vi "FRCts20_WebMethods_S3Upload.vi"(8 "error in (no error)":errorcluster, 9 "Bucket":string, 10 "Object Path":string, 11 "Temporary URL":string) -> (0 "error out":errorcluster)   [LabVIEW 2014, in "FRCts20_Backend_Engine.lvlib"]
uses:
  Backend/source/VI Source/FRCts20_Backend_Engine.lvlib
  <vilib>/National Instruments/NI Amazon Web Services (AWS) Toolkit for LabVIEW/S3/vi source/Typedefs/AMZ_S3_AWS Credentials.ctl
  <vilib>/National Instruments/NI Amazon Web Services (AWS) Toolkit for LabVIEW/S3/vi source/Typedefs/AMZ_S3_API_POST Multipart Object Request Parameters.ctl
  <vilib>/National Instruments/NI Amazon Web Services (AWS) Toolkit for LabVIEW/S3/vi source/Typedefs/AMZ_S3_ACL.ctl
  <vilib>/National Instruments/NI Amazon Web Services (AWS) Toolkit for LabVIEW/S3/vi source/Typedefs/AMZ_S3_Storage Class.ctl
  <vilib>/National Instruments/NI Amazon Web Services (AWS) Toolkit for LabVIEW/S3/vi source/Typedefs/AMZ_S3_Object Metadata.ctl
  <vilib>/National Instruments/NI Amazon Web Services (AWS) Toolkit for LabVIEW/S3/vi source/LV Interface for Amazon S3.lvlib
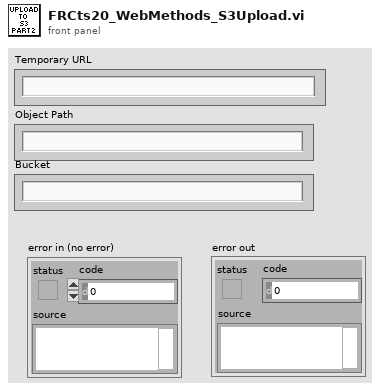
[diagram p1: front panel]
types:
  T1 = typedef "LV Interface for Amazon S3.lvlib/AMZ_S3_API_POST Multipart Object Request Parameters.ctl" = cluster{"Content Type":string, "ACL":T2, "Storage Class":T3, "User Metadata":T4[]}
  T2 = typedef "LV Interface for Amazon S3.lvlib/AMZ_S3_ACL.ctl" = enum16{"private", "public-read", "public-read-write", "authenticated-read", "bucket-owner-read", "bucket-owner-full-control"}
  T3 = typedef "LV Interface for Amazon S3.lvlib/AMZ_S3_Storage Class.ctl" = enum16{"STANDARD", "REDUCED_REDUNDANCY"}
  T4 = typedef "LV Interface for Amazon S3.lvlib/AMZ_S3_Object Metadata.ctl" = cluster{"Key":string, "Value":string}
  T5 = typedef "LV Interface for Amazon S3.lvlib/AMZ_S3_AWS Credentials.ctl" = cluster{"Access Key":string, "Secret Key":string}
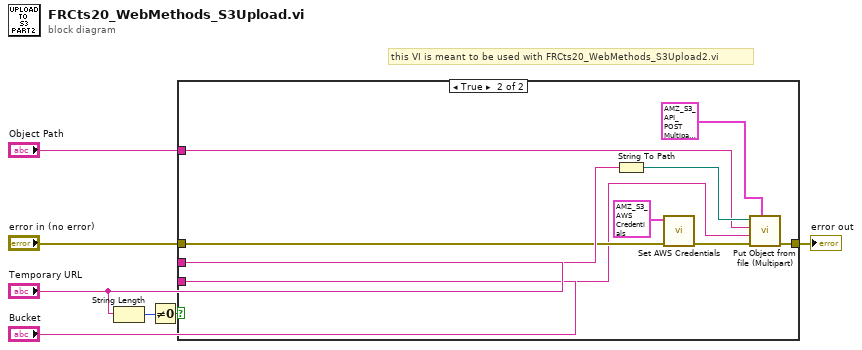
[diagram p0: block diagram]
diagram:
  # "this VI is meant to be used with FRCts20_WebMethods_S3Upload2.vi"
  n1 = String Length(string="Temporary URL") -> (length=w4:i32)
  n2 = Not Equal To 0?(x=w4) -> (x != 0?=w1:bool)
  n3 = case shown="True" w1 {
    tunnel: [w8 w17] -> w7
    tunnel: "Temporary URL" -> [_ w16]
    tunnel: "Object Path" -> [_ w10]
    tunnel: "error in (no error)" -> [w8 w11]
    tunnel: "Bucket" -> [_ w9]
    frame False {
    }
    frame True {
      n4 = String To Path(string=w16) -> (path=w13:path)
      n5 = call <vilib>:"Set AWS Credentials.vi"("error in (no error)"=w11, "AWS Credentials in"=T5 {"Access Key"="AKIAIBWID7GQA3ZVLBGQ", "Secret Key"="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"}) -> ("error out"=w15:errorcluster)  [unwired: 9 in]
      n6 = call <vilib>:"Put Object from file (Multipart).vi"("Request Parameters"=T1 {"Content Type"="binary/octet-stream", "ACL"=enum."public-read", "Storage Class"=enum."REDUCED_REDUNDANCY", "User Metadata"=[]}, "error in (no error)"=w15, "Bucket"=w9, "Object path"=w10, "Local file path"=w13) -> ("error out"=w17:errorcluster)  [unwired: 4 in, 2 out]
    }
  }
  "error out" <- w7
